vi "ZPL Write Read Instrument.vi"(7 "Language":i16=-1 caption="Com Lang (-1 no lang change)" min=-1 max=1, 8 "error in":errorcluster, 9 "Write Command/Query GEN":string, 10 "Write Command/Query SCPI":string, 11 "VISA":refnum<visa-resource-name>) -> (0 "error out":errorcluster, 2 "Response":string, 3 "VISA  out":refnum<visa-resource-name>)   [LabVIEW 2016]
doc: "This VI sends any SCPI or GEN command to the Z+ power supply \n\nIf command returns error (from the instrument's SYST:ERR queue), the VI path, command string and SYST:ERR message are added to the \"error out\" string.\n\nThis VI sends any SCPI or GEN query to the Z+ and reads the response message. The Return Count is the number of characters read.\n\nIf a query error occurs, such as no response message because the query is illegal, the system error (SYST:ERR?) is read and returned in the \"error out\" cluster"
panel:
  out "Unit Address":string
  out "Last EOS":string
  # "Write and Read any Query and Command"
  # "Lambda ZPLUS \n  DC Power Supplies"
  # "Includes error checking\n    after query sent\nAdds checksum to qry string"
  # ")"
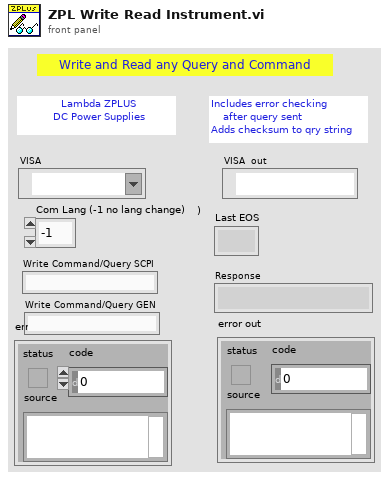
[diagram p1: front panel]
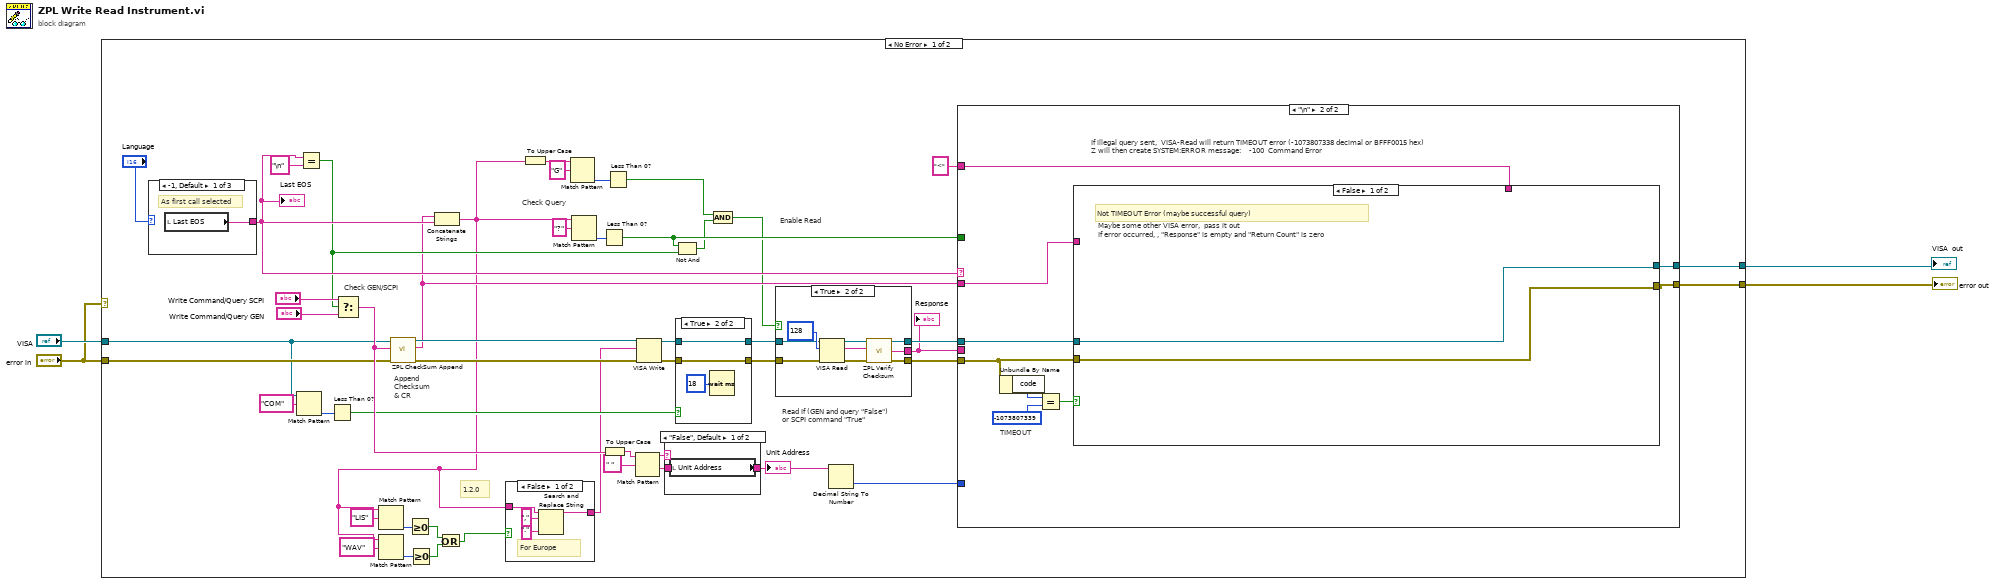
[diagram p0: block diagram]
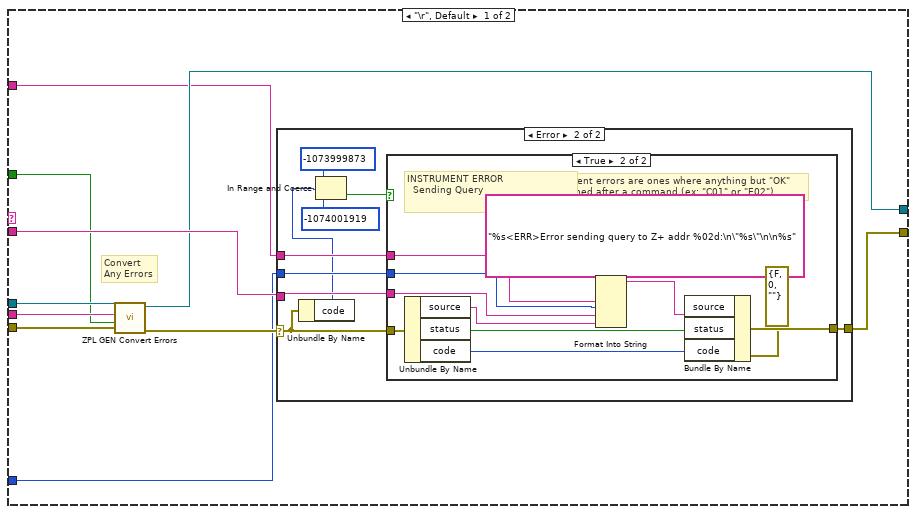
[diagram p5: hidden frame]
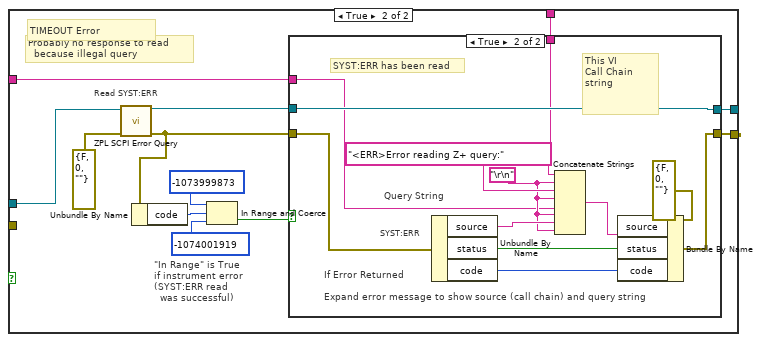
[diagram p8: hidden frame]
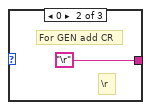
[diagram p10: hidden frame]
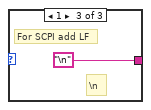
[diagram p11: hidden frame]
diagram:
  n1 = case shown="No Error" "error in" {
    tunnel: "VISA" -> [w16 w149]
    tunnel: [w48 w149] -> w3
    tunnel: [w47 w150] -> w2
    tunnel: "error in" -> [w22 w150]
    frame No Error {
      # "1.2.0"
      # "Append\nChecksum \n& CR"
      # "Enable Read"
      # "Check GEN/SCPI"
      # "Check Query"
      # "Read If (GEN and query \"False\")\nor SCPI command \"True\""
      n2 = case shown="-1, Default" "Language" {
        tunnel: [w135 "\r" "\n"] -> w42
        frame -1, Default {
          # "As first call selected"
          n3 = local read "Last EOS"() -> (w135:string)
        }
        frame 0 {
          # "\\r"
          # "For GEN add CR"
        }
        frame 1 {
          # "\\n"
          # "For SCPI add LF"
        }
      }
      "Last EOS" <- w42
      n4 = Match Pattern(string=w16, regular expression="COM") -> (offset past match=w15:i32)  [unwired: 1 in, 3 out]
      n5 = Equal?(x=w42, y="\n" ("Last EOS 2")) -> (x = y?=w34:bool)
      n6 = Less Than 0?(x=w15) -> (x < 0?=w14:bool)
      n7 = Select(t="Write Command/Query SCPI", s=w34, f="Write Command/Query GEN") -> (s? t:f=w30:string)
      n8 = call "ZPL CheckSum Append.vi"("error"=w22, "Input Cmd"=w30, "VISA"=w16) -> ("error out"=w49:errorcluster, "ChkSum Cmd"=w29:string, "VISA out"=w50:refnum<visa-resource-name>)  [unwired: 6 in]
      n9 = Concatenate Strings(w29, w42) -> (w6:string)
      n10 = Match Pattern(string=w6, regular expression="LIS") -> (offset past match=w10:i32)  [unwired: 1 in, 3 out]
      n11 = Match Pattern(string=w6, regular expression="WAV") -> (offset past match=w9:i32)  [unwired: 1 in, 3 out]
      n12 = Greater Or Equal To 0?(x=w10) -> (x >= 0?=w8:bool)
      n13 = Greater Or Equal To 0?(x=w9) -> (x >= 0?=w7:bool)
      n14 = Or(x=w8, y=w7) -> (x .or. y?=w5:bool)
      n15 = case shown="False" w5 {
        tunnel: w6 -> [w55 w58]
        tunnel: [w54 w58] -> w13
        frame False {
          # "For Europe"
          n16 = Search and Replace String(input string=w55, search string=",", replace string="." ("replace string (\"\")")) -> (result string=w54:string)  [unwired: 5 in, 3 out]
        }
        frame True {
        }
      }
      n17 = To Upper Case(1:w6) -> (0:w27:string)
      n18 = Match Pattern(string=w27, regular expression="G") -> (offset past match=w26:i32)  [unwired: 1 in, 3 out]
      n19 = Match Pattern(string=w6, regular expression="?") -> (offset past match=w52:i32)  [unwired: 1 in, 3 out]
      n20 = Less Than 0?(x=w52) -> (x < 0?=w35:bool)
      n21 = To Upper Case(1:w30) -> (0:w41:string)
      n22 = Less Than 0?(x=w26) -> (x < 0?=w25:bool)
      n23 = Match Pattern(string=w41, regular expression=" ") -> (before substring=w39:string, after substring=w38:string)  [unwired: 1 in, 2 out]
      n24 = VISA Write(VISA resource name=w50, write buffer=w13, error in (no error)=w49) -> (VISA resource name out=w19:refnum<visa-resource-name>, error out=w21:errorcluster)  [unwired: 1 out]
      n25 = case shown="\"False\", Default" w39 {
        tunnel: w38 -> [_ w65]
        tunnel: [w64 w65] -> w37
        frame "False", Default {
          n26 = local read "Unit Address"() -> (w64:string)
        }
        frame "ADR", "INST:NSEL" {
        }
      }
      "Unit Address" <- w37
      n27 = Not And(1:w34, 2:w35) -> (0:w24:bool)
      n28 = case shown="True" w14 {
        tunnel: w21 -> [w59 w62]
        tunnel: [w59 w62] -> w20
        tunnel: w19 -> [w60 w61]
        tunnel: [w60 w61] -> w18
        frame False {
        }
        frame True {
          n29 = Wait (ms)(milliseconds to wait=u32 18) -> ()  [unwired: 1 out]
        }
      }
      n30 = And(x=w25, y=w24) -> (x .and. y?=w23:bool)
      n31 = case shown="True" w23 {
        tunnel: w20 -> [w138 w147]
        tunnel: w18 -> [w139 w146]
        tunnel: [w139 w141] -> w33
        tunnel: [w138 w140] -> w32
        tunnel: [_ w142] -> w31
        frame False {
        }
        frame True {
          n32 = VISA Read(VISA resource name=w146, byte count=u32 128 ("byte count (0)"), error in (no error)=w147) -> (VISA resource name out=w145:refnum<visa-resource-name>, read buffer=w143:string, error out=w144:errorcluster)  [unwired: 1 out]
          n33 = call "ZPL Verify Checksum.vi"("error"=w144, "Input Cmd"=w143, "VISA"=w145) -> ("error out"=w140:errorcluster, "Trimmed String"=w142:string, "VISA out"=w141:refnum<visa-resource-name>)  [unwired: 4 in]
        }
      }
      "Response" <- w31
      n34 = Decimal String To Number(string=w37) -> (number=w36:i32)  [unwired: 2 in, 1 out]
      n35 = case shown="\"\\n\"" w42 {
        tunnel: w32 -> [w74 w103]
        tunnel: w33 -> [w72 w102]
        tunnel: w29 -> [w71 w101]
        tunnel: [w70 w100] -> w48
        tunnel: [w69 w99] -> w47
        tunnel: w31 -> [w75 _]
        tunnel: "<" -> [w68 w98]
        tunnel: w36 -> [w67 _]
        tunnel: w35 -> [w66 _]
        frame "\r", Default {
          # "Convert\nAny Errors"
          n36 = call "ZPL GEN Convert Errors.vi"("error"=w74, "Expect \"OK\" (F)"=w66, "String in"=w75, "VISA"=w72) -> ("error out"=w73:errorcluster, "VISA out"=w70:refnum<visa-resource-name>)  [unwired: 6 in]
          n37 = case shown="Error" w73 {
            selector: w73 -> [w76 w79]
            tunnel: w71 -> [_ w84]
            tunnel: [w76 w85] -> w69
            tunnel: w68 -> [_ w83]
            tunnel: w67 -> [_ w82]
            frame No Error {
              # "Query Sent Correctly \n  and response Returned"
            }
            frame Error {
              n38 = Unbundle By Name(w79) -> ("code"=w78:i32)
              n39 = In Range and Coerce(upper limit=-1073999873 ("code"), x=w78, lower limit=-1074001919 ("code")) -> (In Range?=w77:bool)  [unwired: 1 out]
              n40 = case shown="True" w77 {
                tunnel: w79 -> [w86 w97]
                tunnel: [w86 w94] -> w85
                tunnel: w84 -> [_ w92]
                tunnel: w83 -> [_ w89]
                tunnel: w82 -> [_ w88]
                frame False {
                  # "VISA  ERROR  \n  Sending Command"
                  # "For VISA error, do not change error message"
                }
                frame True {
                  # "Instrument errors are ones where anything but \"OK\"\nis returned after a command (ex: \"C01\" or \"E02\")"
                  # "INSTRUMENT ERROR  \n  Sending Query"
                  n41 = Unbundle By Name(w97) -> ("source"=w91:string, "status"=w95:bool, "code"=w96:i32)
                  n42 = Format Into String(format string="%s<ERR>Error sending query to Z+ addr %02d:\n\"%s\"\n\n%s" ("Source"), w89, w88, w92, w91) -> (resulting string=w90:string)  [unwired: 2 in, 1 out]
                  n43 = Bundle By Name(cluster=errorcluster {"status"=FALSE, "code"=0, "source"=""} ("error out 2"), "source"=w90, "status"=w95, "code"=w96) -> (w94:errorcluster)
                }
              }
            }
          }
        }
        frame "\n" {
          # "TIMEOUT"
          # "If illegal query sent,  VISA-Read will return TIMEOUT error (-1073807338 decimal or BFFF0015 hex) \nZ will then create SYSTEM:ERROR message:    -100  Command Error"
          n44 = Unbundle By Name(w103) -> ("code"=w104:i32)
          n45 = Equal?(x=w104, y=-1073807339 ("code")) -> (x = y?=w106:bool)
          n46 = case shown="False" w106 {
            tunnel: [w107 w119] -> w99
            tunnel: [w108 w120] -> w100
            tunnel: w102 -> [w108 w110]
            tunnel: w103 -> [w107 _]
            tunnel: w101 -> [_ w111]
            tunnel: w98 -> [_ w109]
            frame False {
              # "Maybe some other VISA error,  pass it out\nIf error occurred, , \"Response\" is empty and \"Return Count\" is zero"
              # "Not TIMEOUT Error (maybe successful query)"
            }
            frame True {
              # "\"In Range\" is True\nif instrument error\n(SYST:ERR read\n  was successful)"
              # "TIMEOUT Error"
              # "Probably no response to read  \n  because illegal query"
              # "Read SYST:ERR"
              n47 = call "ZPL SCPI Error Query.vi"("error"=errorcluster {"status"=FALSE, "code"=0, "source"=""}, "VISA"=w110) -> ("error out"=w113:errorcluster, "VISA out"=w112:refnum<visa-resource-name>)  [unwired: 6 in, 2 out]
              n48 = Unbundle By Name(w113) -> ("code"=w115:i32)
              n49 = In Range and Coerce(upper limit=-1073999873 ("code"), x=w115, lower limit=-1074001919 ("code")) -> (In Range?=w116:bool)  [unwired: 1 out]
              n50 = case shown="True" w116 {
                tunnel: w113 -> [w122 w128]
                tunnel: [w122 w129] -> w119
                tunnel: w112 -> [w121 w127]
                tunnel: [w121 w127] -> w120
                tunnel: w111 -> [_ w125]
                tunnel: w109 -> [_ w123]
                frame False {
                  # "Read SYST:ERR returned VISA communication error.\n  Comm is dead,  just pass error out"
                }
                frame True {
                  w126 = "\r\n"
                  # "This VI \nCall Chain \nstring"
                  # "Query String"
                  # "Expand error message to show source (call chain) and query string"
                  # "SYST:ERR"
                  # "If Error Returned"
                  # "SYST:ERR has been read"
                  n51 = Unbundle By Name(w128) -> ("source"=w131:string, "status"=w133:bool, "code"=w132:i32)
                  n52 = Concatenate Strings(w123, w126, "<ERR>Error reading Z+ query:" ("Source"), w126, w125, w126, w131, w126) -> (w134:string)
                  n53 = Bundle By Name(cluster=errorcluster {"status"=FALSE, "code"=0, "source"=""} ("error out 2"), "source"=w134, "status"=w133, "code"=w132) -> (w129:errorcluster)
                }
              }
            }
          }
        }
      }
    }
    frame Error {
    }
  }
  "VISA  out" <- w3
  "error out" <- w2
